vi "Set Number Of Steps.vi"(11 "Manual Mode Command in":refnum<class "Manual Mode Command.lvclass">) -> (3 "Manual Mode Command out":refnum<class "Manual Mode Command.lvclass">)   [LabVIEW 2016, in "Manual Mode Command.lvclass"]
uses:
  Manual Mode Command.lvclass
  Manual Mode Command.lvclass/Manual Mode Command.ctl
panel:
  in  "Number Of Steps":i32
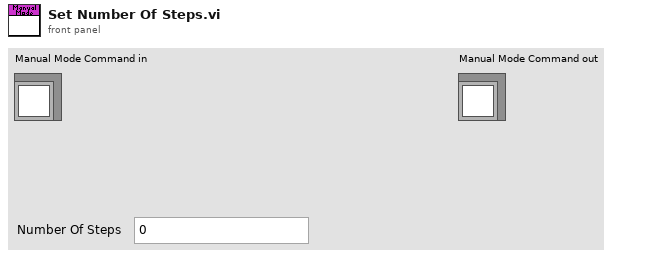
[diagram p1: front panel]
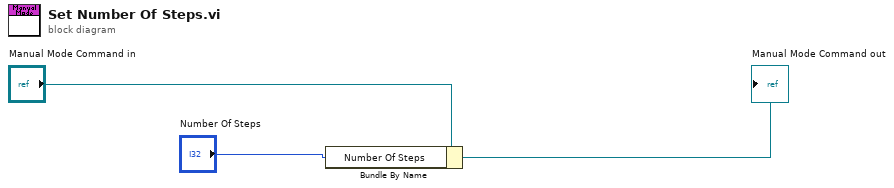
[diagram p0: block diagram]
diagram:
  n1 = Bundle By Name(cluster="Manual Mode Command in", "Number Of Steps"="Number Of Steps") -> (→"Manual Mode Command out":refnum<class "Manual Mode Command.lvclass">)
